vi "HoppingStep(Nonlinear-XZ-TargetBaselineDefer).vi"() -> ()   [LabVIEW 2014]
uses:
  <vilib>/Platform/TimedLoop/XDataNode/timing_clust.ctl
  <vilib>/Platform/TimedLoop/XDataNode/nitl_modes.ctl
  <vilib>/Platform/TimedLoop/XDataNode/wakeup.ctl
  <vilib>/rvi/Emulation/niFpgaGetClockAttributes.vi
  <vilib>/rvi/Emulation/niFpgaSctlEmulationGetInTimedLoop.vi
  <vilib>/rvi/Emulation/niFpgaEmulationReportErrorSimple.vi
  <vilib>/rvi/Emulation/niFpgaProcessEmulError.vi
  <vilib>/rvi/eio/common/nirviEmuTemplateMethod_errors.vi
  <vilib>/rvi/Emulation/niFpgaCriticalErrorInLSC.vi
  <vilib>/rvi/interface/RandomDataEmulation/niFpgaRandomDataHandleErrors.vi
  <vilib>/eio/EIONode/EIONode.xnode
  <vilib>/Platform/TimedLoop/XDataNode/XDataNode.xnode
  <vilib>/rvi/DataTransferAndStorage/Container/XNode/niFpgaContainer.xnode
  <vilib>/rvi/interface/RandomDataEmulation/nirviRandomDataFpgaReadWriteTemplate.vi
  <vilib>/Platform/TimedLoop/XDataNode/XDNodeRunTimeDep.lvlib
panel:
  in  "BaselineDeferMultiplier":u32
  in  "ScanLayerNum":u32
  in  "threshold":sgl
  in  "ExtraStepIn":u32
  in  "TimeConstant":u32
  in  "LowPassFilter":i16
  in  "BottomSleep us":i16=80
  in  "UpperSleep us":i16=150
  out "ZRealPos":i16
  in  "RelativeWithdraw":i16
  out "Waveform Chart":i32(graph)
  in  "stop":bool
  out "Z":i32(graph)
  in  "ZOffset":i16
  in  "XOffset":i16
  in  "XNum":i16
  in  "XStepIndex":i16
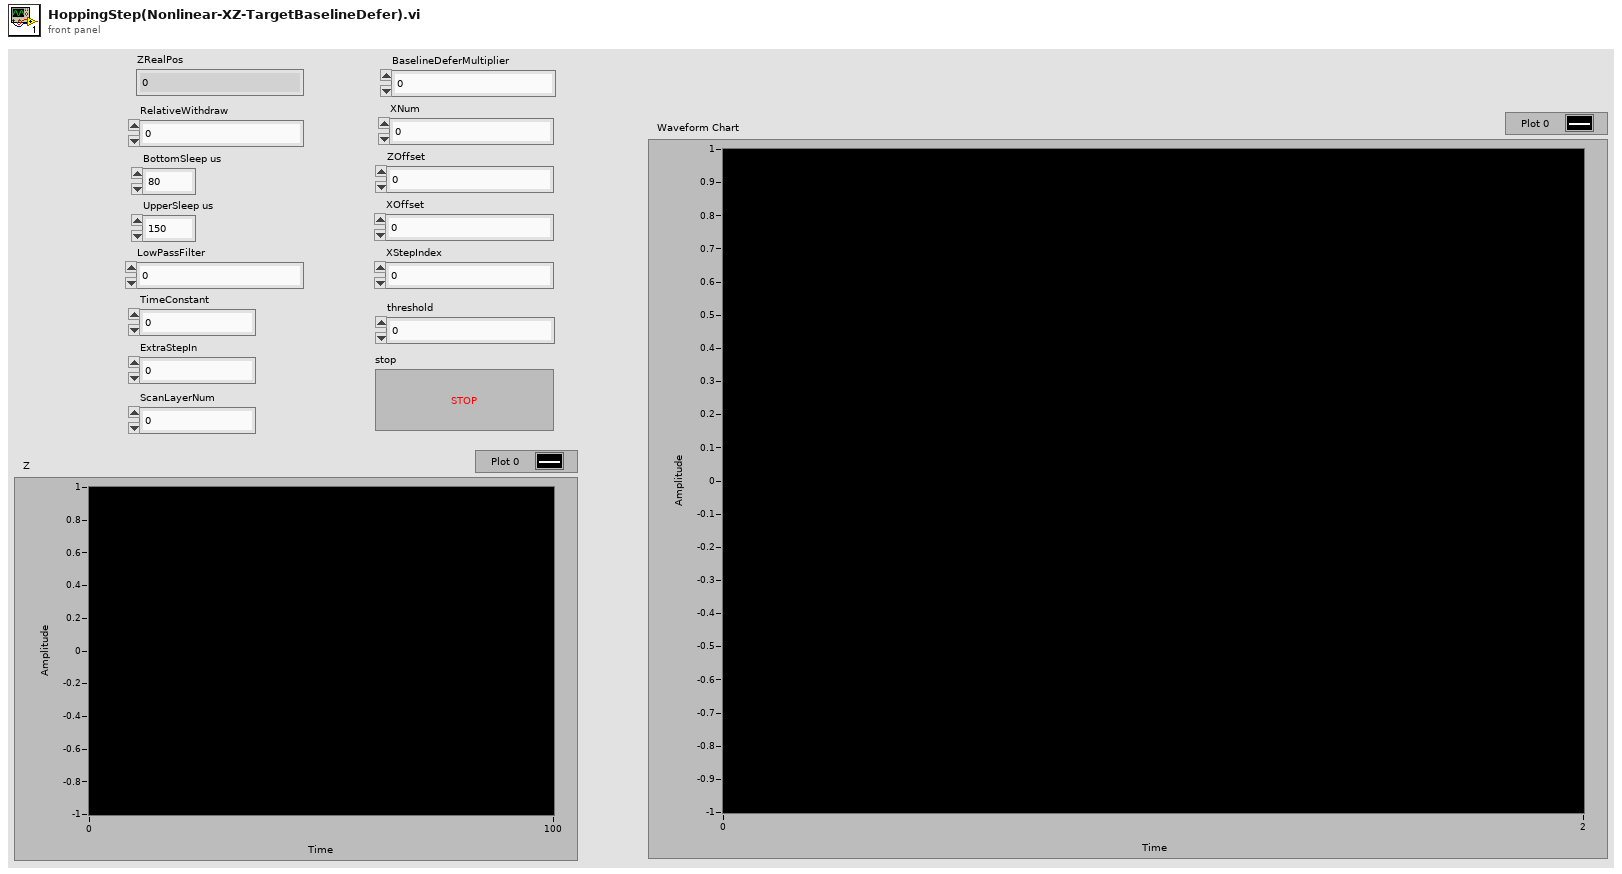
[diagram p1: front panel]
types:
  T1 = typedef "XDNodeRunTimeDep.lvlib/timing_clust.ctl" = cluster{"Expected End [f-1]":u64, "Actual End [f-1]":u64, "Finished Late? [f-1]":bool, "Expected End [i-1]":u64, "Actual End [i-1]":u64, "Finished Late? [i-1]":bool, "Expected Start [i]":u64, "Actual Start [i]":u64, "Expected Start [f]":u64, "Actual Start [f]":u64, "Source Name":string, "Structure Name":string, "Period":i64, "Deadline":i64, "Offset":i64, "Start":i64, "Priority":i32, "Timeout":i32, "Mode":T2, "Wakeup Reason":T3, "Error":errorcluster, "Source Type":string, "Secondary Source Type":string, "Global End Time":u64, "Global Start Time":u64, "Frame Duration":u64, "Iteration Duration":u64, "Assigned CPU":i32, "I/O Scan Engine Mode":u32}
  T2 = typedef "XDNodeRunTimeDep.lvlib/nitl_modes.ctl" = enum32{"No Change", "Process missed periods, maintain original phase", "Discard missed periods, maintain original phase", "Process missed periods, ignore original phase", "Discard missed periods, ignore original phase"}
  T3 = typedef "XDNodeRunTimeDep.lvlib/wakeup.ctl" = enum32{"Normal", "Aborted", "Asynchronous wakeup", "Timing source error", "Timed loop error", "Timeout"}
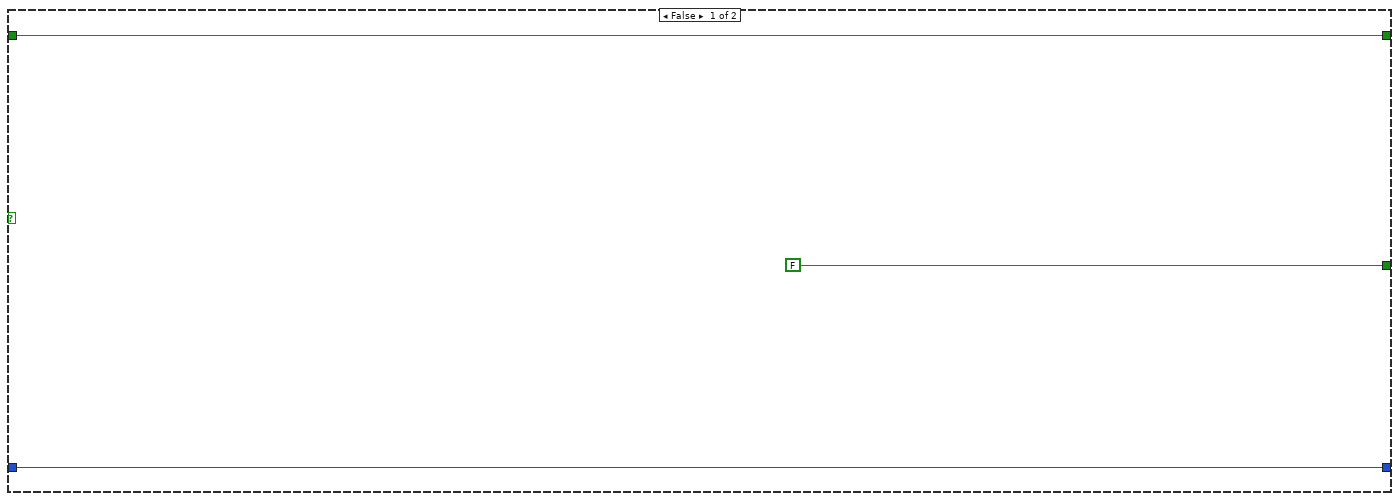
[diagram p3: hidden frame]
diagram:
  n1 = flat-sequence {
    frame #0 {
      n2 = call "Wait"("Count(mSec)"=u32 100 ("Count(uSec)")) -> ()  [unwired: 1 out]
    }
    frame #1 {
      w2 = i16 0
      n3 = local write "RelativeWithdraw"("RelativeWithdraw") -> ()
      n4 = local write "TimeConstant"("TimeConstant") -> ()
      n5 = local write "ExtraStepIn"("ExtraStepIn") -> ()
      n6 = local write "BottomSleep us"("BottomSleep us") -> ()
      n7 = local write "UpperSleep us"("UpperSleep us") -> ()
      n8 = local write "LowPassFilter"("LowPassFilter") -> ()
      n9 = local write "ScanLayerNum"("ScanLayerNum") -> ()
      n10 = local write "BaselineDeferMultiplier"("BaselineDeferMultiplier") -> ()
      n11 = local write "threshold"("threshold") -> ()
      n12 = while {
        tunnel: "XNum" -> [w49]
        tunnel: "XStepIndex" -> [w50]
        shift-right: [w40] -> _
        shift-left: "ZOffset" -> [w51]
        tunnel: "XOffset" -> [w47]
        shift-right: [w21] -> _
        shift-left: w2 -> [w29]
        shift-right: [w18] -> _
        shift-left: w2 -> [w26]
        i -> [w30]
        stop <- w53 stop-if-true
        # "X step loop"
        n13 = Decrement(x=w49) -> (x-1=w48:i16)
        n14 = Multiply(x=w50, y=w30) -> (x*y=w52:i32)
        n15 = Greater Or Equal?(x=w30, y=w48) -> (x >= y?=w45:bool)
        n16 = Add(x=w47, y=w52) -> (x+y=w42:i32)
        n17 = flat-sequence {
          tunnel: [w55] -> w46
          tunnel: w51 -> [w55]
          tunnel: w45 -> [w64]
          tunnel: [w64] -> w44
          tunnel: w42 -> [w63]
          tunnel: w30 -> [w62]
          tunnel: [w62] -> w39
          tunnel: w30 -> [w57]
          tunnel: w29 -> [w61]
          tunnel: [w61] -> w27
          tunnel: w26 -> [w60]
          tunnel: [w60] -> w24
          tunnel: [w56] -> w16
          tunnel: [w71] -> w38
          tunnel: w46 -> [w71]
          tunnel: [w70] -> w36
          tunnel: w44 -> [w70]
          tunnel: [w69] -> w34
          tunnel: w39 -> [w69]
          tunnel: [w67] -> w28
          tunnel: w27 -> [w67]
          tunnel: [w66] -> w25
          tunnel: w24 -> [w66]
          tunnel: [w65] -> w17
          tunnel: w16 -> [w65]
          tunnel: w38 -> [w73]
          tunnel: [w73] -> w37
          tunnel: w36 -> [w79]
          tunnel: [w79] -> w35
          tunnel: w34 -> [w78]
          tunnel: [w78] -> w33
          tunnel: [w75] -> w32
          tunnel: [w74] -> w31
          tunnel: w28 -> [w77]
          tunnel: w25 -> [w76]
          tunnel: [w75] -> w23
          tunnel: [w74] -> w22
          tunnel: w17 -> [w72]
          tunnel: w37 -> [w104]
          tunnel: [w103] -> w54
          tunnel: w35 -> [w102]
          tunnel: [w102] -> w43
          tunnel: [w101] -> w41
          tunnel: w33 -> [w100]
          tunnel: w32 -> [w99]
          tunnel: w31 -> [w98]
          tunnel: w23 -> [w97]
          tunnel: w22 -> [w96]
          tunnel: [w97] -> w20
          tunnel: [w96] -> w19
          tunnel: [w351] -> w40
          tunnel: [w352] -> w53
          tunnel: w41 -> [w351]
          tunnel: w43 -> [w348]
          tunnel: w54 -> [w349]
          tunnel: [w347] -> w21
          tunnel: w20 -> [w347]
          tunnel: w19 -> [w346]
          tunnel: [w346] -> w18
          frame #0 {
            n18 = local read "BaselineDeferMultiplier"() -> (w58:u32)
            n19 = Quotient & Remainder(x=w57, y=w58) -> (x-y*floor(x/y)=w59:u32)  [unwired: 1 out]
            n20 = xnode "FPGA I/O Node"("Connector0/AO2"=w63, "Connector0/AO0"=w55) -> ()  [unwired: 2 in, 2 out]
            n21 = Equal To 0?(x=w59) -> (x = 0?=w56:bool)
          }
          frame #1 {
            n22 = call "Wait3"("Count(mSec)"=u32 2) -> ()  [unwired: 1 out]
          }
          frame #2 {
            n23 = case shown="True" w72 {
              tunnel: [w81 w90] -> w75
              tunnel: [w80 w89] -> w74
              tunnel: w77 -> [w81 _]
              tunnel: w76 -> [w80 _]
              frame False {
              }
              frame True {
                # "Threshold deviation"
                # "Reference current"
                n24 = for {
                  N: 32 -> [_]
                  shift-right: [w95] -> w87
                  shift-left: 0 -> [w94]
                  n25 = local read "TimeConstant"() -> (w91:u32)
                  n26 = xnode "FPGA I/O Node"() -> ("Connector0/AI1"=w92:i16)  [unwired: 1 in, 1 out]
                  n27 = To Long Integer(number=w92) -> (32bit integer=w93:i32)
                  n28 = Add(x=w93, y=w94) -> (x+y=w95:i32)
                  n29 = call "Wait2"("Count(uSec)"=w91) -> ()  [unwired: 1 out]
                }
                n30 = local read "threshold"() -> (w85:sgl)
                n31 = Logical Shift(y=i8 -5, x=w87) -> (x << y=w88:i32)
                n32 = Multiply(x=w85, y=w88) -> (x*y=w83:sgl)
                n33 = To Word Integer(number=w83) -> (16bit integer=w89:i16)
                n34 = To Word Integer(number=w88) -> (16bit integer=w90:i16)
              }
            }
          }
          frame #3 {
            n35 = while {
              tunnel: [w120] -> w103
              shift-right: [w117] -> w101
              shift-left: w104 -> [w121]
              tunnel: w100 -> [w112]
              tunnel: w99 -> [w106]
              tunnel: w98 -> [w105]
              i -> [w116]
              stop <- w113 stop-if-true
              n36 = flat-sequence {
                tunnel: [w126] -> w124
                tunnel: [w125] -> w123
                tunnel: [w129] -> w122
                tunnel: w121 -> [w129]
                tunnel: w116 -> [w128]
                tunnel: [w128] -> w115
                tunnel: w112 -> [w127]
                tunnel: [w127] -> w111
                tunnel: w106 -> [w126]
                tunnel: w105 -> [w125]
                tunnel: w124 -> [w135]
                tunnel: w123 -> [w134]
                tunnel: w122 -> [w133]
                tunnel: [w136] -> w119
                tunnel: [w132] -> w118
                tunnel: w115 -> [w131]
                tunnel: [w131] -> w114
                tunnel: w111 -> [w130]
                tunnel: [w130] -> w110
                tunnel: w119 -> [w336]
                tunnel: w118 -> [w338]
                tunnel: w114 -> [w332]
                tunnel: w110 -> [_]
                tunnel: [w336] -> w109
                tunnel: [w340] -> w108
                tunnel: [w337] -> w107
                tunnel: [w343] -> w113
                tunnel: [w344] -> w117
                tunnel: [w345] -> w120
                tunnel: w109 -> [w345]
                tunnel: w108 -> [w344]
                tunnel: w107 -> [w343]
                frame #0 {
                }
                frame #1 {
                  n37 = while {
                    tunnel: [w146] -> w136
                    tunnel: w135 -> [w152]
                    tunnel: w134 -> [w151]
                    shift-right: [w148] -> _
                    shift-left: w133 -> [w149]
                    tunnel: [w140] -> w132
                    i -> [w143]
                    stop <- w147 stop-if-true
                    n38 = Equal To 0?(x=w143) -> (x = 0?=w144:bool)
                    n39 = while {
                      tunnel: w152 -> [w188]
                      tunnel: w151 -> [w189]
                      tunnel: ["stop"] -> w157
                      shift-right: [w172] -> w140
                      shift-left: w149 -> [w185]
                      tunnel: i16 300 -> [w174]
                      tunnel: [w171] -> w161
                      tunnel: [w170] -> w160
                      tunnel: w144 -> [w169]
                      i -> [w173]
                      stop <- w191 stop-if-true
                      n40 = flat-sequence {
                        tunnel: w189 -> [w207]
                        tunnel: w188 -> [w205]
                        tunnel: w185 -> [w203]
                        tunnel: w174 -> [w199]
                        tunnel: w173 -> [w198]
                        tunnel: w169 -> [w195]
                        tunnel: [w204] -> w168
                        tunnel: [w202] -> w167
                        tunnel: [w201] -> w166
                        tunnel: [w197] -> w165
                        tunnel: [w196] -> w164
                        tunnel: [w237] -> w170
                        tunnel: [w238] -> w171
                        tunnel: [w239] -> w175
                        tunnel: [w240] -> w184
                        tunnel: [w241] -> w186
                        tunnel: w168 -> [w241]
                        tunnel: w167 -> [w240]
                        tunnel: w166 -> [w239]
                        tunnel: w165 -> [w238]
                        tunnel: w164 -> [w237]
                        frame #0 {
                          n41 = xnode "FPGA I/O Node"() -> ("Connector0/AI1"=w206:i16)  [unwired: 1 in, 1 out]
                          n42 = Negate(x=w198) -> (-x=w200:i32)
                          n43 = Scale By Power Of 2(n=w200, x=w199) -> (x*2^n=w194:i16)
                          n44 = Select(t=w194, s=w195, f=i16 1) -> (s? t:f=w192:i16)
                          n45 = node-c288(refnum<k21> "40 MHz Onboard Clock" ("Source Name")) -> (w210:T1)
                          n46 = timed-loop {
                            timing: w210 -> [_]
                            timing-out: [_] -> w209
                            tunnel: w205 -> [w228]
                            tunnel: w207 -> [w212]
                            tunnel: w206 -> [w211]
                            tunnel: [w224] -> w204
                            tunnel: [w223] -> w202
                            tunnel: w203 -> [w213]
                            tunnel: w192 -> [w216]
                            tunnel: [w218] -> w201
                            tunnel: w198 -> [w218]
                            tunnel: [w212] -> w196
                            tunnel: [w211] -> w197
                            stop <- TRUE stop-if-true
                            # "Range excess judgement"
                            n47 = Subtract(x=w211, y=w228) -> (x-y=w214:i16)
                            n48 = Greater?(x=w216, y=i16 2) -> (0:w215:bool)
                            n49 = Absolute Value(x=w214) -> (abs(x)=w227:i16)
                            n50 = Greater Or Equal?(x=w213, y=i16 29000) -> (x >= y?=w225:bool)
                            n51 = Select(t=w216, s=w215, f=1) -> (s? t:f=w219:i32)
                            n52 = Greater Or Equal?(x=w227, y=w212) -> (x >= y?=w226:bool)
                            n53 = Or(x=w226, y=w225) -> (x .or. y?=w223:bool)
                            n54 = Add(x=w219, y=w213) -> (x+y=w221:i32)
                            n55 = Select(t=w213, s=w223, f=w221) -> (s? t:f=w224:i32)
                          }
                          n56 = node-c288(w209) -> ()
                        }
                        frame #1 {
                          n57 = call "Wait11"("Count(uSec)"=u32 50) -> ()  [unwired: 1 out]
                        }
                      }
                      n58 = flat-sequence {
                        tunnel: [w246] -> w187
                        tunnel: w186 -> [w246]
                        tunnel: w184 -> [w245]
                        tunnel: [w245] -> w183
                        tunnel: [w243] -> w176
                        tunnel: w175 -> [w244]
                        tunnel: w187 -> [w247]
                        tunnel: [w247] -> w182
                        tunnel: w183 -> [w252]
                        tunnel: [w252] -> w180
                        tunnel: [w250] -> w177
                        tunnel: w176 -> [w249]
                        tunnel: w182 -> [w255]
                        tunnel: [w255] -> w181
                        tunnel: w180 -> [w254]
                        tunnel: [w254] -> w179
                        tunnel: [w253] -> w178
                        tunnel: w177 -> [w253]
                        tunnel: w181 -> [w257]
                        tunnel: [w257] -> w172
                        tunnel: w178 -> [w256]
                        frame #0 {
                          n59 = local read "BottomSleep us"() -> (w242:i16)
                          n60 = Add(x=w244, y=w242) -> (x+y=w243:i32)
                        }
                        frame #1 {
                          n61 = local read "UpperSleep us"() -> (w248:i16)
                          n62 = xnode "FPGA I/O Node"("Connector0/AO0"=w247) -> ()  [unwired: 1 in, 1 out]
                          n63 = Greater?(x=w249, y=w248) -> (0:w251:bool)
                          n64 = Select(t=w248, s=w251, f=w249) -> (s? t:f=w250:i32)
                        }
                        frame #2 {
                        }
                        frame #3 {
                          n65 = call "Wait10"("Count(uSec)"=w256) -> ()  [unwired: 1 out]
                        }
                      }
                      n66 = Or(x=w179, y="stop") -> (x .or. y?=w191:bool)
                      "Z" <- w172
                    }
                    n67 = for {
                      N: 4 -> [_]
                      tunnel: w157 -> [w263]
                      tunnel: [w263] -> w162
                      shift-right: [w259] -> w139
                      shift-left: 0 -> [w261]
                      n68 = xnode "FPGA I/O Node"() -> ("Connector0/AI1"=w262:i16)  [unwired: 1 in, 1 out]
                      n69 = local read "TimeConstant"() -> (w258:u32)
                      n70 = call "Loop Timer2"("Count(uSec)"=w258) -> ()  [unwired: 1 out]
                      n71 = To Long Integer(number=w262) -> (32bit integer=w260:i32)
                      n72 = Add(x=w260, y=w261) -> (x+y=w259:i32)
                    }
                    n73 = Logical Shift(y=i8 -2, x=w139) -> (x << y=w138:i32)
                    n74 = Subtract(x=w138, y=w161) -> (x-y=w156:i32)
                    n75 = Absolute Value(x=w156) -> (abs(x)=w155:i32)
                    n76 = Greater Or Equal?(x=w155, y=w160) -> (x >= y?=w154:bool)
                    n77 = Not(x=w162) -> (.not. x?=w153:bool)
                    n78 = And(x=w153, y=w154) -> (x .and. y?=w163:bool)
                    n79 = case shown="True" w163 {
                      tunnel: w162 -> [w266 w273]
                      tunnel: [w266 w272] -> w146
                      tunnel: w161 -> [_ w271]
                      tunnel: w160 -> [_ w270]
                      tunnel: w140 -> [w265 w269]
                      tunnel: [w265 w268] -> w148
                      tunnel: [FALSE w267] -> w145
                      frame False {
                      }
                      frame True {
                        n80 = while {
                          tunnel: w271 -> [w282]
                          tunnel: w270 -> [w281]
                          tunnel: [w278] -> w267
                          shift-right: [w279] -> w268
                          shift-left: w269 -> [w280]
                          tunnel: w273 -> [w284]
                          tunnel: [w283] -> w272
                          i -> [w276]
                          stop <- w274 stop-if-true
                          n81 = flat-sequence {
                            tunnel: w281 -> [w300]
                            tunnel: w282 -> [w301]
                            tunnel: w284 -> [w302]
                            tunnel: [w302] -> w292
                            tunnel: [w301] -> w291
                            tunnel: [w300] -> w290
                            tunnel: w280 -> [w294]
                            tunnel: [w293] -> w289
                            tunnel: [w299] -> w277
                            tunnel: w276 -> [w299]
                            tunnel: [w308] -> w288
                            tunnel: [w307] -> w287
                            tunnel: [w306] -> w286
                            tunnel: w292 -> [w308]
                            tunnel: w291 -> [w307]
                            tunnel: w290 -> [w306]
                            tunnel: [w305] -> w285
                            tunnel: w289 -> [w305]
                            tunnel: w277 -> [w303]
                            tunnel: [w303] -> w275
                            tunnel: w288 -> [w326]
                            tunnel: [w326] -> w283
                            tunnel: w287 -> [w321]
                            tunnel: w286 -> [w320]
                            tunnel: w285 -> [w319]
                            tunnel: [w319] -> w279
                            tunnel: [w313] -> w278
                            tunnel: w275 -> [w318]
                            tunnel: [w314] -> w274
                            frame #0 {
                              n82 = Quotient & Remainder(x=w299, y=4) -> (x-y*floor(x/y)=w297:i32)  [unwired: 1 out]
                              n83 = Equal To 0?(x=w297) -> (x = 0?=w296:bool)
                              n84 = Increment(x=w294) -> (x+1=w295:i32)
                              n85 = Select(t=w295, s=w296, f=w294) -> (s? t:f=w293:i32)
                              n86 = xnode "FPGA I/O Node"("Connector0/AO0"=w293) -> ()  [unwired: 1 in, 1 out]
                            }
                            frame #1 {
                              n87 = local read "TimeConstant"() -> (w304:u32)
                              n88 = call "Wait6"("Count(uSec)"=w304) -> ()  [unwired: 1 out]
                            }
                            frame #2 {
                              n89 = for {
                                N: 4 -> [_]
                                shift-right: [w328] -> w310
                                shift-left: 0 -> [w330]
                                n90 = xnode "FPGA I/O Node"() -> ("Connector0/AI1"=w331:i16)  [unwired: 1 in, 1 out]
                                n91 = local read "TimeConstant"() -> (w327:u32)
                                n92 = To Long Integer(number=w331) -> (32bit integer=w329:i32)
                                n93 = Add(x=w329, y=w330) -> (x+y=w328:i32)
                                n94 = call "Wait5"("Count(uSec)"=w327) -> ()  [unwired: 1 out]
                              }
                              n95 = local read "ExtraStepIn"() -> (w317:u32)
                              n96 = Decrement(x=w317) -> (x-1=w316:u32)
                              n97 = Logical Shift(y=i8 -2, x=w310) -> (x << y=w309:i32)
                              n98 = Greater Or Equal?(x=w318, y=w316) -> (x >= y?=w315:bool)
                              n99 = Subtract(x=w309, y=w321) -> (x-y=w323:i32)
                              n100 = Absolute Value(x=w323) -> (abs(x)=w322:i32)
                              n101 = Greater Or Equal?(x=w322, y=w320) -> (x >= y?=w313:bool)
                              n102 = Not(x=w313) -> (.not. x?=w312:bool)
                              n103 = Or(x=w312, y=w315) -> (x .or. y?=w314:bool)
                            }
                          }
                        }
                      }
                    }
                    n104 = Greater Or Equal?(x=w143, y=40) -> (x >= y?=w141:bool)
                    n105 = Compound Arithmetic op=OR(w146, w145, w141) -> (w147:bool)
                  }
                }
                frame #2 {
                  n106 = local read "RelativeWithdraw"() -> (w341:i16)
                  n107 = local read "ScanLayerNum"() -> (w334:u32)
                  n108 = Decrement(x=w334) -> (x-1=w333:u32)
                  n109 = Subtract(x=w338, y=w341) -> (x-y=w340:i32)
                  n110 = Greater Or Equal?(x=w332, y=w333) -> (x >= y?=w335:bool)
                  n111 = xnode "FPGA I/O Node"("Connector0/AO0"=w340) -> ()  [unwired: 1 in, 1 out]
                  n112 = xnode ("FIFO Method Node")("Element"=w338, "Timeout"=0) -> ()  [unwired: 1 in, 2 out]
                  n113 = Or(x=w336, y=w335) -> (x .or. y?=w337:bool)
                  "Waveform Chart" <- w338
                  "ZRealPos" <- w338
                }
                frame #3 {
                  n114 = call "Wait7"("Count(mSec)"=u32 2) -> ()  [unwired: 1 out]
                }
              }
            }
          }
          frame #4 {
            n115 = Or(x=w349, y=w348) -> (x .or. y?=w352:bool)
            n116 = call "Wait4"("Count(mSec)"=u32 1) -> ()  [unwired: 1 out]
          }
        }
      }
    }
    frame #2 {
      n117 = xnode "FPGA I/O Node"("Connector0/AO0"=i16 0) -> ()  [unwired: 1 in, 1 out]
    }
    frame #3 {
      n118 = call "Wait8"("Count(uSec)"=u32 200) -> ()  [unwired: 1 out]
    }
    frame #4 {
      n119 = local read "XOffset"() -> (w355:i16)
      n120 = xnode "FPGA I/O Node"("Connector0/AO2"=w355) -> ()  [unwired: 1 in, 1 out]
    }
    frame #5 {
      n121 = call "Wait9"("Count(uSec)"=u32 400) -> ()  [unwired: 1 out]
    }
  }
